vi "Apply Speed.vi"(8 "error in (no error)":errorcluster, 11 "Tool Rectangle in":refnum<class "Tool Rectangle.lvclass">) -> (0 "error out":errorcluster, 3 "Tool Rectangle out":refnum<class "Tool Rectangle.lvclass">)   [LabVIEW 2019, in "Tool Rectangle.lvclass"]
uses:
  Tool Rectangle.lvclass
  Settings/ObjectSettings/ObjectSettings.lvclass/ObjectSettings.ctl
  Settings/Rectangle Settings/Rectangle Settings.lvclass
  C:/Users/Albro/Documents/GitHub/AFM-Lithography/lvsrc/Classes/Settings/ObjectSettings/ObjectSettings.lvclass
  Settings/ObjectSettings/ObjectSettings.lvclass
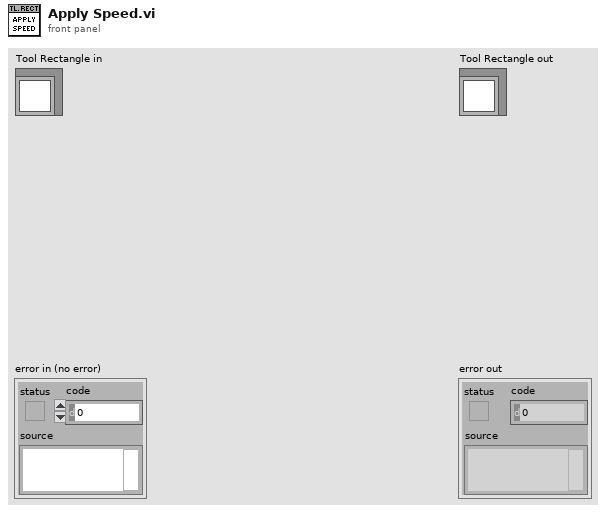
[diagram p1: front panel]
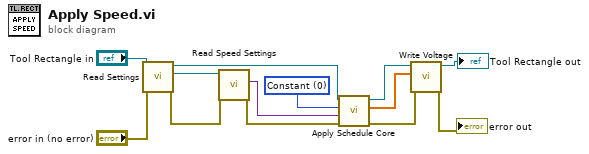
[diagram p0: block diagram]
diagram:
  w3 = u16 0 items=["Constant", "Ramp", "Function", "Formula"] ("Schedule")
  n1 = call-dynamic "Read Settings.vi"("error in (no error)"="error in (no error)", "Tool Rectangle in"="Tool Rectangle in") -> ("error out"=w5:errorcluster, "Rectangle Settings.lvclass"=w7:refnum<class "Rectangle Settings.lvclass">, "Tool Rectangle out"=w10:refnum<class "Tool Rectangle.lvclass">)  [unwired: 7 in]
  n2 = call "Read Speed Settings.vi"("error in (no error)"=w5, "ObjectSettings in"=w7) -> ("error out"=w4:errorcluster, "Settings"=w6:variant)  [unwired: 7 in, 1 out]
  n3 = call-dynamic "Apply Schedule Core.vi"("error in (no error)"=w4, "Settings"=w6, "Schedule"=w3, "Tool Object in"=w10) -> ("error out"=w13:errorcluster, "Schedule Array"=w11:dbl[], "Tool Object out"=w12:refnum<class "Tool Rectangle.lvclass">)  [unwired: 5 in]
  n4 = call-dynamic "Write Voltage.vi"("error in (no error)"=w13, "Voltage"=w11, "Tool Object in"=w12) -> ("error out"=→"error out":errorcluster, "Tool Object out"=→"Tool Rectangle out":refnum<class "Tool Rectangle.lvclass">)  [unwired: 7 in]
